vi "Read Name.vi"(8 "error in (no error)":errorcluster, 11 "INode in":refnum<class "INode.lvclass">) -> (0 "error out":errorcluster, 2 "Name":string, 3 "INode out":refnum<class "INode.lvclass">)   [LabVIEW 2023, in "d7.lvlib" / "INode.lvclass"]
uses:
  INode.lvclass
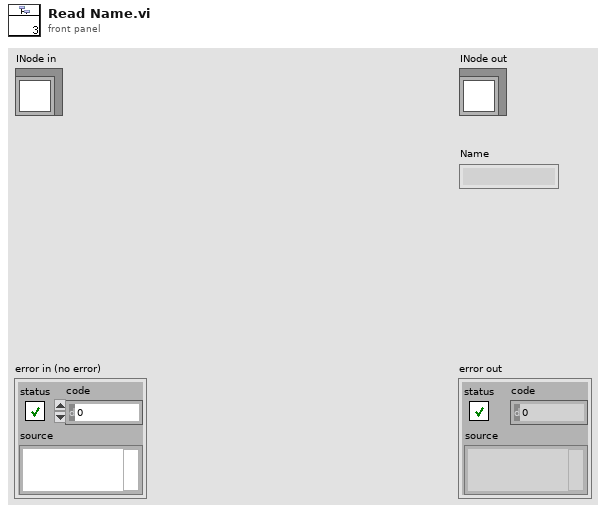
[diagram p1: front panel]
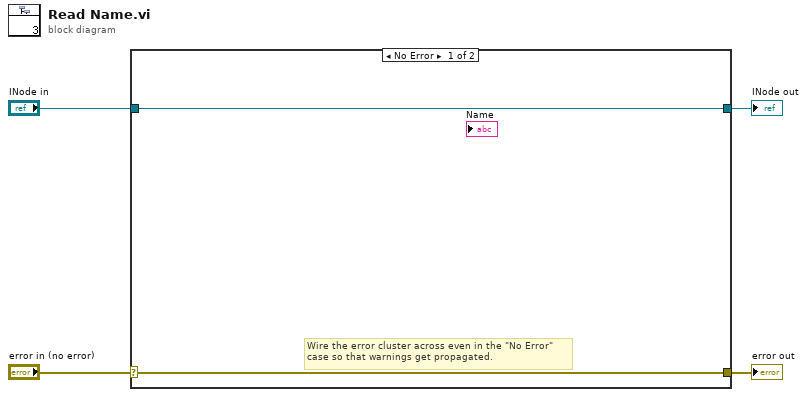
[diagram p0: block diagram]
diagram:
  n1 = case shown="No Error" "error in (no error)" {
    selector: "error in (no error)" -> [w5 w8]
    tunnel: [w5 w8] -> w3
    tunnel: [w6 w7] -> w1
    tunnel: "INode in" -> [w6 w7]
    frame No Error {
      # "Wire the error cluster across even in the \"No Error\"\ncase so that warnings get propagated."
    }
    frame Error {
    }
  }
  "error out" <- w3
  "INode out" <- w1
